vi "Dashboard Main.vi"() -> ()   [LabVIEW 2023]
uses:
  <vilib>/event_ctls.llb/eventvkey.ctl
  <vilib>/Rock Robotics/Network Tables/NT Read Numeric Array.vi
  <vilib>/Rock Robotics/Network Tables/NT Read Boolean.vi
  <vilib>/Rock Robotics/WPI/Dashboard/WPI_DashboardLogging Global.vi
panel:
  in  "Camera Settings Right":T1={"Frame Rate"=30, "Compression"=30, "Size"=1, "DB Camera Config"=FALSE} {"Frame Rate" scale=1.0..30.0; "Compression" scale=100.0..-1.0; "Size" items=["640x480", "320x240", "160x120"]}
  in  "Camera Name Right":string(combo)="No Camera Selection"
  out "Camera Perf":string
  in  "Camera Settings":T1={"Frame Rate"=30, "Compression"=30, "Size"=1, "DB Camera Config"=FALSE} {"Frame Rate" scale=1.0..30.0; "Compression" scale=100.0..-1.0; "Size" items=["640x480", "320x240", "160x120"]}
  in  "TCP":refnum<k5>
  in  "Rec Mode":enum32{"Stop", "Record", "Playback"}(radio)
  out "Robot IP":string
  out "Image Message":string="Timeout in Camera Communications"
  in  "Dashboard Tab":T2(tab)
  in  "Select Auto":string(combo)="Select Autonomous ..."
  out "NT Connection":bool
  out "MotorChart R":cluster{"Numeric":dbl, "Numeric":dbl}(graph)
  out "MotorChart L":cluster{"Numeric":dbl, "Numeric":dbl}(graph)
  out "MotorSliders R":cluster{"MotorSlide1":dbl, "MotorSlide2":dbl} {"MotorSlide2" scale=-1.0..1.0 scale format="%#_2e"; "MotorSlide1" scale=-1.0..1.0 scale format="%#_2e"}
  out "MotorSliders L":cluster{"MotorSlide1":dbl, "MotorSlide2":dbl} {"MotorSlide2" scale=-1.0..1.0 scale format="%#_2e"; "MotorSlide1" scale=-1.0..1.0 scale format="%#_2e"}
  out "Gyro":dbl(knob) scale=0.0..360.0
  out "JS1 Z":dbl(slide) scale=-1.0..1.0 scale format="%#_2e"
  out "JS1 Graph":cluster{"X":dbl, "Y":dbl}[](graph)
  out "JS1 Buttons":T3
  out "JS2 Z":dbl(slide) scale=-1.0..1.0 scale format="%#_2e"
  out "JS2 Graph":cluster{"X":dbl, "Y":dbl}[](graph)
  out "JS2 Buttons":T3
  out "Mode":T4(ring)=enum."Auto Disabled"
  out "Right Camera Perf":cluster{"Bandwidth (Mbps)":dbl, "FPS":dbl}
  out "Camera Image Right":T5(plugin-control)
  in  "DB/String 9":string
  in  "DB/String 8":string
  in  "DB/String 7":string
  in  "DB/String 6":string
  in  "DB/String 5":string
  in  "DB/String 4":string
  in  "DB/String 3":string
  in  "DB/String 2":string
  in  "DB/String 1":string
  in  "DB/String 0":string
  in  "DB/Slider 0":dbl(slide) scale=0.0..5.0
  in  "DB/Slider 1":dbl(slide) scale=0.0..5.0
  in  "DB/Slider 2":dbl(slide) scale=0.0..5.0
  in  "DB/Slider 3":dbl(slide) scale=0.0..5.0
  out "DB/LED 3":bool
  out "DB/LED 2":bool
  out "DB/LED 1":bool
  out "DB/LED 0":bool
  in  "DB/Button 3":bool
  in  "DB/Button 2":bool
  in  "DB/Button 1":bool
  in  "DB/Button 0":bool caption="New Name"
  out "Shoot Motor Out R":dbl format="%14.3f"
  out "Shoot PV RPM R":dbl format="%14.0f"
  in  "Shoot  SP RPM":dbl min=-5000.0 max=5000.0 step=200.0 format="%14.0f"
  out "Shoot Control R":T6(graph)
  out "Shoot Speed On Targ L":bool
  out "Shoot Speed On Targ R":bool
  out "Shoot PV RPM L":dbl format="%14.0f"
  out "Shoot Motor Out L":dbl format="%14.3f"
  out "Intake Motor Out":dbl format="%14.3f"
  out "Intake PV RPM":dbl format="%14.0f"
  in  "Intake  SP PCT":dbl min=-1.0 max=1.0 step=0.05 format="%14.3f"
  out "Intake Control":T7(graph)
  in  "Test Slider":dbl(slide) scale=0.0..100.0 scale format="%#_3g"
  in  "On/Off":bool caption="Solenoid"
  in  "Test Name":u16(ring) items=["Select the test to run..."]
  in  "Test Tree":string(tree)
  in  "Motor":cluster{"Value":dbl, "Enable":bool} {"Value" scale=-1.0..1.0 scale format="%#_3g"}
  out "Progress":T8 {"Test Progress" scale=0.0..100.0}
  in  "Rev/Fwd":cluster{"Forward":bool, "Reverse":bool}
  in  "Test Ring":u16(ring) items=["Monochrome", "Color"]
  in  "CheckList":i32(listbox)
  out "Tree":string(tree)
  out "Camera Image":T5(plugin-control)
  out "Background":bool
  in  "Camera Name":string(combo)="No Camera Selection"
  # "HW"
  # "HW"
  # "Joysticks"
  # "Drive Motors"
  # "Front"
  # "Right"
  # "Left"
  # "Back"
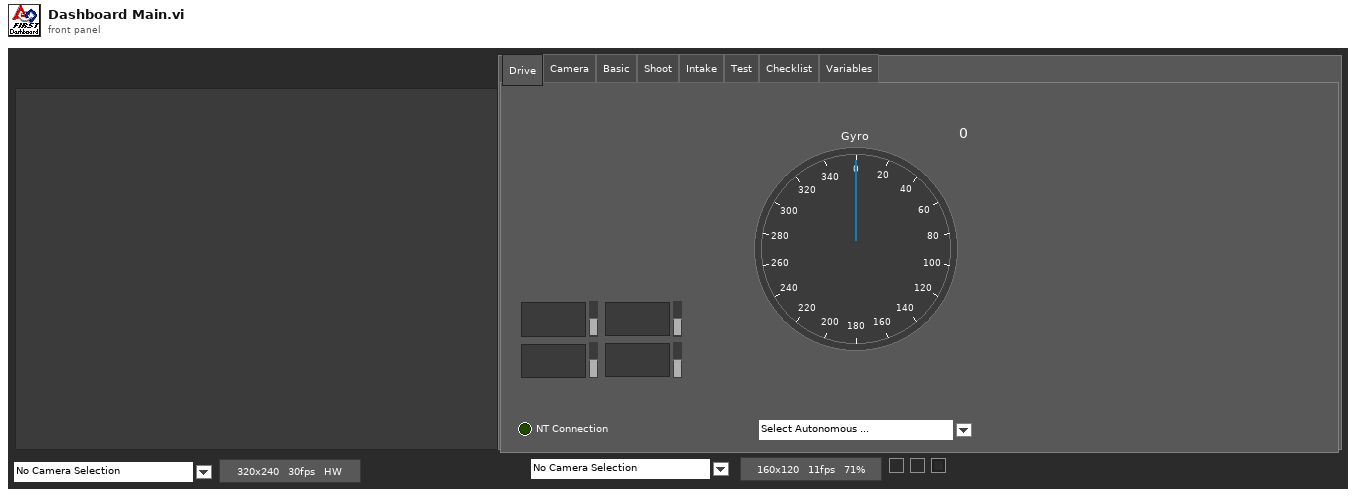
[diagram p1: front panel]
types:
  T1 = cluster{"Frame Rate":i32, "Compression":i32, "Size":u16, "DB Camera Config":bool}
  T2 = enum32{"Drive", "Camera", "Basic", "Shoot", "Intake", "Test", "Checklist", "Variables"}
  T3 = cluster{bool, bool, bool, bool, bool, bool, bool, bool, bool, bool, bool, bool}
  T4 = enum8{"Tele-Op Disabled", "Tele-Op Enabled", "Auto Disabled", "Auto Enabled", "Test Disabled", "Test Enabled", "Disconnected", "No Code", "E-Stop"}
  T5 = typedef "IMAQ Image.ctl" = refnum<image>
  T6 = cluster{"Setpoint":dbl, "FeedForward":dbl, "CO-ControlOutput":dbl, "Velocity_RPM":dbl}
  T7 = cluster{"Intake  SP PCT":dbl, "value":dbl, "value":dbl, "value":dbl}
  T8 = cluster{"Test Progress":u8, "Test Progress Text":string}
  T9 = cluster{"Save Path":path, "Interval (s)":dbl, "Keep":i32}
  T10 = enum32{"Drive", "Camera", "Basic", "Custom", "Test", "Commands", "Checklist", "Variables"}
  T11 = typedef "Image Type" = u32
  T12 = cluster{"Error Strings":string, "Disable Counts":cluster{u16, u16}, "Rail Faults":cluster{u16, u16, u16}, "Robot IP":string, "DB Mode":u8, "Event Info":cluster{"Name":string, "Type":u8, "Number":u16, "Replay":u8}}
  T13 = cluster{"Storage":cluster{"Disk Free":u64, "RAM Block":u32, "RAM free":u32}, "CPU Utilization":cluster{"CPU % ISR":sgl, "CPU % Time Crit":sgl, "CPU % Timed Str":sgl, "CPU % High":sgl, "CPU % Above":sgl, "CPU % Normal":sgl, "CPU % Low":sgl}, "CAN":cluster{"% Bus Utilization":sgl, "Bus Off Cnt":u32, "TX_FIFO Full Cnt":u32, "Receive Error Cnt":u8, "Transmit Error Cnt":u8}, "HID":cluster{"HID Outputs":u32, "Rumble Low":u16, "Rumble High":u16}[]}
  T14 = cluster{"Status bits":cluster{"Test Mode":bool, "Autonomous":bool, "Enabled":bool, "Code Start":bool, "Brownout":bool, "Reserved 2":bool, "Reserved 3":bool, "E-Stop":bool}, "Code Trace":cluster{"Disabled":bool, "TeleOp":bool, "Auto":bool, "Test":bool}, "Controller Type":enum16{"unknown", "cRIO", "roboRio"}, "Code?":enum16{"unknown", "noCode", "code"}, "Battery V":dbl}
  T15 = cluster{"Control Bits":cluster{"TestMode":bool, "Autonomous":bool, "Enabled":bool, "FMS Present":bool, bool, bool, bool, "E-Stop":bool}, "Team Station ":u8, "Countdown":sgl, "Joystick Values":cluster{"Axes":dbl[], "Buttons":bool[], "POVs":i16[]}[]}
  T16 = cluster{"Axes":dbl[], "Buttons":bool[], "POVs":i16[]}[]
  T17 = cluster{"Axes":dbl[], "Buttons":bool[], "POVs":i16[]}
  T18 = cluster{"Buttons[0]":bool, "Buttons[1]":bool, "Buttons[2]":bool, "Buttons[3]":bool, "Buttons[4]":bool, "Buttons[5]":bool, "Buttons[6]":bool, "Buttons[7]":bool, "Buttons[8]":bool, "Buttons[9]":bool, "Buttons[10]":bool, "Buttons[11]":bool}
  T19 = cluster{"Intake  SP PCT":dbl, dbl, "value":dbl, "value":dbl}
  T20 = cluster{"Shoot  SP RPM":dbl, "value":dbl, "value":dbl, "value":dbl}
  T21 = cluster{"Camera Image":refnum<vi>, "Dashboard Tab":refnum<vi>, "Background":refnum<vi>, "Rec Mode":refnum<vi>, "Test Slider":refnum<vi>, "On/Off ":refnum<vi>, "Test Ring":refnum<vi>, "Rev/Fwd":refnum<vi>, "Test Name":refnum<vi>, "Motor":refnum<vi>, "Progress":refnum<vi>, "CheckList":refnum<vi>, "Tree":refnum<vi>, "Test Tree":refnum<vi>, "Camera Settings":refnum<vi>, "Camera Name":refnum<vi>, "Camera Perf":refnum<vi>, "Camera Settings Right":refnum<vi>, "Camera Name Right":refnum<vi>, "Camera Image Right":refnum<vi>}
  T22 = cluster{"Global Rectangle":i32[], "Contours":cluster{"Contour Type":u32, "ROI Type":u32, "Points":i32[]}[]}
  T23 = cluster{"Camera Name":string, string, "Saved DB Images Info":cluster{"Save Path":path, "Interval (s)":dbl, "Keep":i32}}
  T24 = cluster{"Camera Name Right":string, string, "Saved DB Images Info":cluster{"Save Path":path, "Interval (s)":dbl, "Keep":i32}}
  T25 = cluster{"Operation":enum16{"Update", "Clear"}, "Color Box":u32}[]
  T26 = typedef "eventvkey.ctl" = enum16{"ASCII", "Enter", "Return", "Shift", "Ctrl", "Alt", "Cmd", "Opt", "Caps", "NumLock", "Clear", "Break", "Up", "Down", "Left", "Right", "Insert", "Delete", "Home", "End", "PageUp", "PageDown", "Escape", "Help", "Pause", "ScrollLock", "F1", "F2", "F3", "F4", "F5", "F6", "F7", "F8", "F9", "F10", "F11", "F12", "F13", "F14", "F15", "F16", "F17", "F18", "F19", "F20", "F21", "F22", "F23", "F24", "Play", "VolumeUp", "VolumeDown", "Mute", "Two Byte Char"}
  T27 = cluster{"Image Size":bool, "Image Type":bool, "Pixel Value":bool, "ROI Information":bool, "Zoom Factor":bool}
  T28 = cluster{"Operation":enum16{"Update", "Clear"}, "Color Box":u32}
  T29 = cluster{"Shift":bool, "Ctrl":bool, "Alt":bool, "Cmd":bool, "Opt":bool}
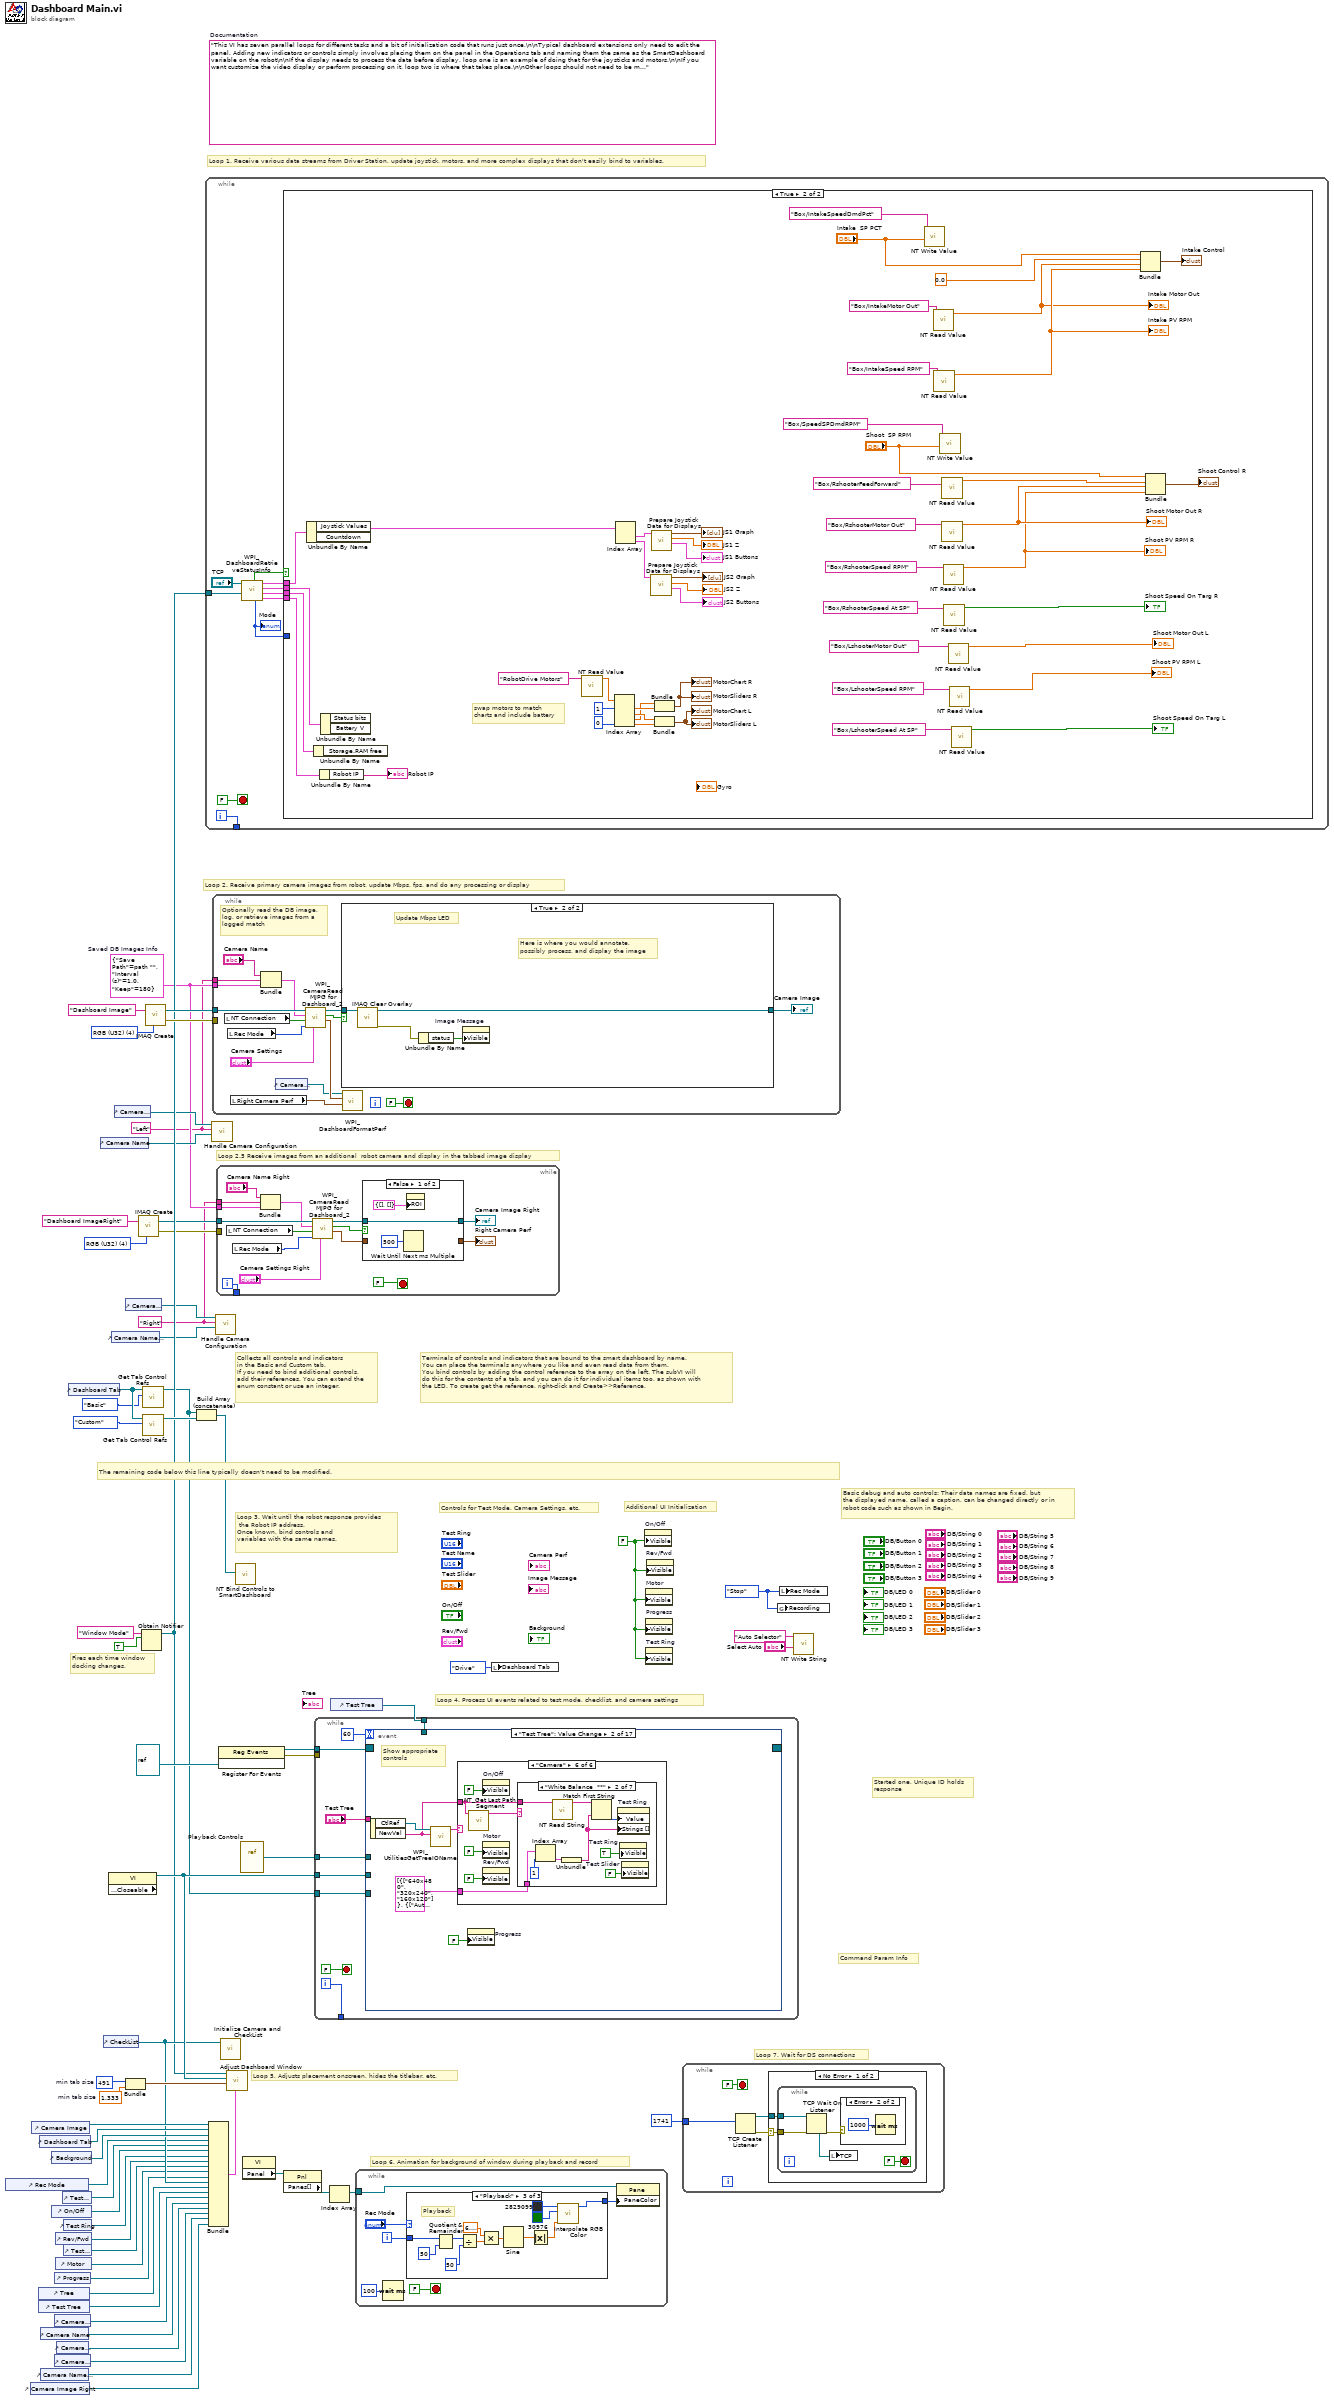
[diagram p0: block diagram]
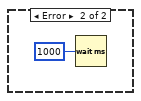
[diagram p4: hidden frame]
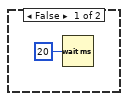
[diagram p5: hidden frame]
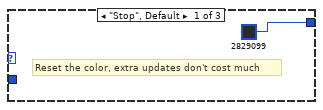
[diagram p6: hidden frame]
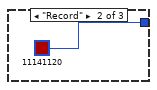
[diagram p7: hidden frame]
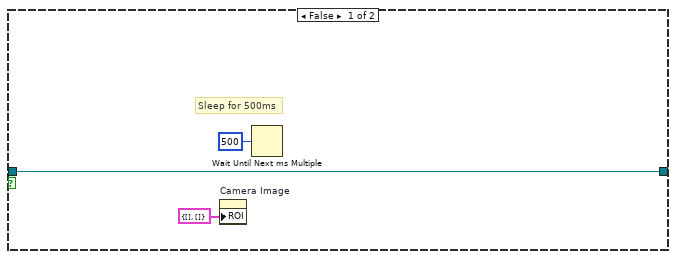
[diagram p8: hidden frame]
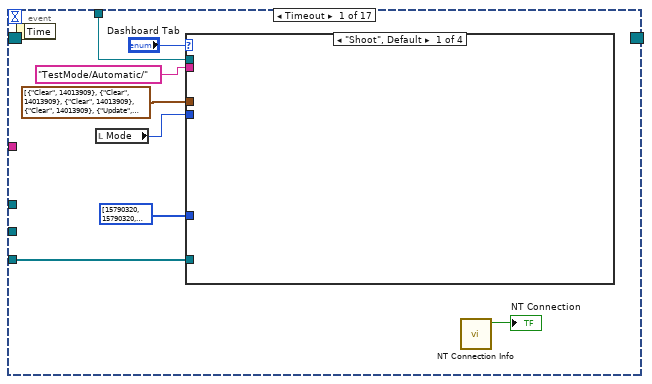
[diagram p9: hidden frame]
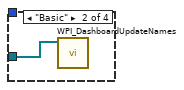
[diagram p10: hidden frame]
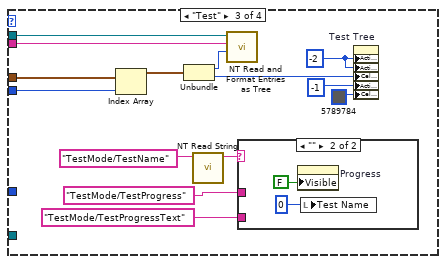
[diagram p11: hidden frame]
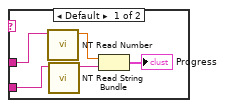
[diagram p12: hidden frame]
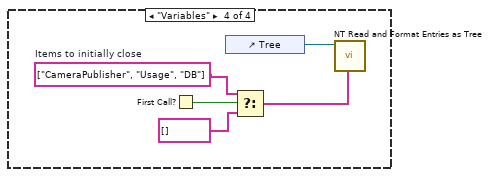
[diagram p13: hidden frame]
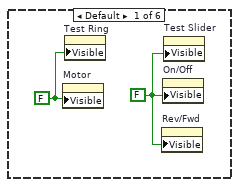
[diagram p14: hidden frame]
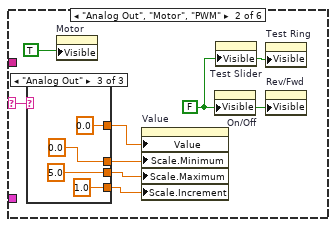
[diagram p15: hidden frame]
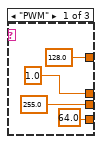
[diagram p16: hidden frame]
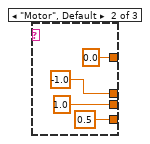
[diagram p17: hidden frame]
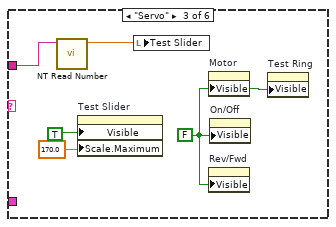
[diagram p18: hidden frame]
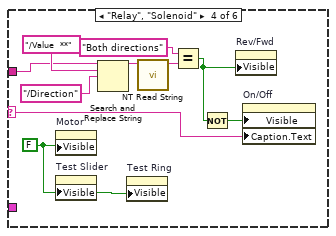
[diagram p19: hidden frame]
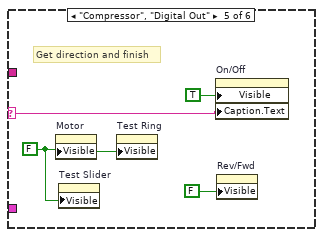
[diagram p20: hidden frame]
diagram:
  w4 = T9 {"Save Path"=path "", "Interval (s)"=1.0, "Keep"=180}  # Saved DB Images Info
  w3 = "Right"
  w2 = "Left"
  w14 = T11 4 items=["Grayscale (U8)", "Grayscale (I16)", "Grayscale (SGL)", "Complex (CSG)", "RGB (U32)", "HSL (U32)", "RGB (U64)"] ("Image Type")
  w42 = 491  # min tab size
  w41 = 1.333  # min tab size
  w49 = enum32{"Stop", "Record", "Playback"}."Stop" ("Rec Mode")
  w26 = FALSE ("Visible")
  (unwired) "This VI has seven parallel loops for different tasks and a bit of initialization code that runs just once.\n\nTypical dashboard extensions only need to edit the panel. Adding new indicators or controls simply involves placing them on the panel in the Operations tab and naming them the same as the SmartDashboard variable on the robot\n\nIf the display needs to process the data before display, loop one is an example of doing that for the joysticks and motors.\n\nIf you want customize the video display or perform processing on it, loop two is where that takes place.\n\nOther loops should not need to be modified. They are pretty standard, and document the task they perform."  # Documentation
  w63 = T11 4 items=["Grayscale (U8)", "Grayscale (I16)", "Grayscale (SGL)", "Complex (CSG)", "RGB (U32)", "HSL (U32)", "RGB (U64)"] ("Image Type")
  # "Loop 2.5 Receive images from an additional  robot camera and display in the tabbed image display"
  # "Command Param Info"
  # "Started one, Unique ID holds\nresponse"
  # "Loop 7. Wait for DS connections"
  # "Basic debug and auto controls: Their data names are fixed, but\nthe displayed name, called a caption, can be changed directly or in\nrobot code such as shown in Begin."
  # "Controls for Test Mode, Camera Settings, etc."
  # "Additional UI Initialization"
  # "Loop 6. Animation for background of window during playback and record"
  # "Fires each time window\ndocking changes."
  # "Collects all controls and indicators\nin the Basic and Custom tab.\nIf you need to bind additional controls,\nadd their references. You can extend the\nenum constant or use an integer."
  # "The remaining code below this line typically doesn't need to be modified."
  # "Loop 4. Process UI events related to test mode, checklist, and camera settings"
  # "Terminals of controls and indicators that are bound to the smart dashboard by name.\nYou can place the terminals anywhere you like and even read data from them.\nYou bind controls by adding the control reference to the array on the left. The subVI will\ndo this for the contents of a tab, and you can do it for individual items too, as shown with\nthe LED. To create get the reference, right-click and Create>>Reference."
  # "Loop 3. Wait until the robot response provides\n the Robot IP address.\nOnce known, bind controls and\nvariables with the same names."
  # "Loop 5. Adjusts placement onscreen, hides the titlebar, etc."
  # "Loop 1. Receive various data streams from Driver Station, update joystick, motors, and more complex displays that don't easily bind to variables."
  # "Loop 2. Receive primary camera images from robot, update Mbps, fps, and do any processing or display"
  n1 = control-ref of="Rec Mode"() -> (w32:refnum<vi>)
  n2 = control-ref of="Camera Image Right"() -> (w7:refnum<vi>)
  n3 = control-ref of="Camera Image"() -> (w44:refnum<vi>)
  n4 = control-ref of="Tree"() -> (w36:refnum<vi>)
  n5 = control-ref of="Test Tree"() -> (w35:refnum<vi>)
  n6 = control-ref of="Dashboard Tab"() -> (w43:refnum<vi>)
  n7 = control-ref of="Camera Name"() -> (w20:refnum<vi>)
  n8 = control-ref of="Camera Name Right"() -> (w8:refnum<vi>)
  n9 = control-ref of="Background"() -> (w39:refnum<vi>)
  n10 = control-ref of="On/Off"() -> (w30:refnum<vi>)
  n11 = control-ref of="Progress"() -> (w27:refnum<vi>)
  n12 = control-ref of="Camera Settings"() -> (w21:refnum<vi>)
  n13 = control-ref of="Camera Settings Right"() -> (w9:refnum<vi>)
  n14 = control-ref of="Rev/Fwd"() -> (w28:refnum<vi>)
  n15 = control-ref of="Motor"() -> (w33:refnum<vi>)
  n16 = control-ref of="Camera Perf"() -> (w19:refnum<vi>)
  n17 = control-ref of="Test Slider"() -> (w31:refnum<vi>)
  n18 = control-ref of="Test Ring"() -> (w29:refnum<vi>)
  n19 = control-ref of="Test Name"() -> (w34:refnum<vi>)
  n20 = control-ref of="Dashboard Tab"() -> (w47:refnum<vi>)
  n21 = control-ref of="Camera Name"() -> (w22:refnum<vi>)
  n22 = control-ref of="CheckList"() -> (w37:refnum<vi>)
  n23 = property class="VI" props=["Front Panel.Closeable"]() -> (reference out=w48:refnum<vi>)  [unwired: 2 in, 2 out]
  n24 = control-ref of="Camera Name Right"() -> (w10:refnum<vi>)
  n25 = control-ref of="Camera Settings"() -> (w23:refnum<vi>)
  n26 = control-ref of="Camera Settings Right"() -> (w11:refnum<vi>)
  n27 = Bundle("min tab size"=w42, "min tab size"=w41) -> (w40:cluster{"min tab size":i32, "min tab size":dbl})  [unwired: 1 in]
  n28 = call "IMAQ Create"("Image Name"="Dashboard ImageRight", "Image Type"=w14) -> ("New Image"=w13:T5, "error out"=w12:errorcluster)  [unwired: 2 in, 1 out]
  n29 = Obtain Notifier(name (unnamed)="Window Mode", notification data type=TRUE) -> (notifier out=w25:refnum<notifier>)  [unwired: 2 in, 2 out]
  n30 = call <vilib>:"Get Tab Control Refs.vi"("Page Index"=T10."Basic" ("Dashboard Tab"), "TabControl in"=w47) -> ("ControlsOnPage"=w18:refnum<vi>[])  [unwired: 9 in]
  n31 = call <vilib>:"Get Tab Control Refs.vi"("Page Index"=T10."Custom" ("Dashboard Tab"), "TabControl in"=w47) -> ("ControlsOnPage"=w46:refnum<vi>[])  [unwired: 9 in]
  n32 = call "IMAQ Create"("Image Name"="Dashboard Image", "Image Type"=w63) -> ("New Image"=w61:T5, "error out"=w60:errorcluster)  [unwired: 2 in, 1 out]
  n33 = Build Array (concatenate)(w18, w46) -> (w45:refnum<vi>[])
  n34 = while {
    tunnel: [w72] -> _
    tunnel: w25 -> [w64]
    i -> [w72]
    stop <- FALSE stop-if-true
    n35 = call <vilib>:"WPI_DashboardRetrieveStatusInfo.vi"("Window Mode Notifier"=w64, "TCP Cnx"="TCP") -> ("Power and Errors"=w67:T12, "Robot Metrics"=w70:T13, "Status Info"=w71:T14, "Control Info"=w68:T15, "Robot Mode"=w66:T4, "Process?"=w69:bool)  [unwired: 4 in]
    "Mode" <- w66
    n36 = case shown="True" w69 {
      tunnel: w71 -> [_ w123]
      tunnel: w70 -> [_ w122]
      tunnel: w68 -> [_ w121]
      tunnel: w67 -> [_ w120]
      tunnel: w66 -> [_ _]
      frame False {
        n37 = Wait (ms)(milliseconds to wait=u32 20) -> ()  [unwired: 1 out]
      }
      frame True {
        # "swap motors to match\ncharts and include battery"
        n38 = Unbundle By Name(w121) -> ("Joystick Values"=w111:T16)  [unwired: 1 out]
        n39 = Unbundle By Name(w122) -> ()  [unwired: 1 out]
        n40 = Unbundle By Name(w120) -> ("Robot IP"=→"Robot IP":string)
        n41 = Unbundle By Name(w123) -> ()  [unwired: 2 out]
        n42 = call-poly <vilib>:"NT Read Value.vi"("name"="RobotDrive Motors" ("Name")) -> ("value"=w101:dbl[])  [unwired: 8 in, 2 out]
        n43 = Index Array(array=w101, index #1=1, index #4=0) -> (element #1=w115:dbl, element #2=w116:dbl, element #3=w114:dbl, element #4=w119:dbl)  [unwired: 2 in]
        n44 = Index Array(array=w111) -> (element #1=w110:T17, element #2=w106:T17)  [unwired: 2 in]
        n45 = call "Prepare Joystick Data for Displays.vi"("Joystick Values"=w106) -> ("Buttons"=→"JS2 Buttons":T18, "Z Axis"=→"JS2 Z":dbl, "Cartesian Data"=→"JS2 Graph":cluster{"X axis":dbl, "X axis":dbl}[])  [unwired: 8 in]
        n46 = call "Prepare Joystick Data for Displays.vi"("Joystick Values"=w110) -> ("Buttons"=→"JS1 Buttons":T18, "Z Axis"=→"JS1 Z":dbl, "Cartesian Data"=→"JS1 Graph":cluster{"X axis":dbl, "X axis":dbl}[])  [unwired: 8 in]
        n47 = Bundle("Numeric"=w114, "Numeric"=w115) -> (→"MotorChart R" →"MotorSliders R":cluster{"Numeric":dbl, "Numeric":dbl})  [unwired: 1 in]
        n48 = Bundle("Numeric"=w116, "Numeric"=w119) -> (→"MotorChart L" →"MotorSliders L":cluster{"Numeric":dbl, "Numeric":dbl})  [unwired: 1 in]
        n49 = call-poly <vilib>:"NT Write Value.vi"("value"="Intake  SP PCT", "name"="Box/IntakeSpeedDmdPct") -> ()  [unwired: 9 in, 1 out]
        n50 = call-poly <vilib>:"NT Read Value.vi"("name"="Box/IntakeMotor Out") -> ("value"=w75:dbl)  [unwired: 8 in, 2 out]
        "Intake Motor Out" <- w75
        n51 = call-poly <vilib>:"NT Read Value.vi"("name"="Box/IntakeSpeed RPM") -> ("value"=w97:dbl)  [unwired: 8 in, 2 out]
        "Intake PV RPM" <- w97
        n52 = call-poly <vilib>:"NT Write Value.vi"("value"="Shoot  SP RPM", "name"="Box/SpeedSPDmdRPM") -> ()  [unwired: 9 in, 1 out]
        n53 = call-poly <vilib>:"NT Read Value.vi"("name"="Box/RshooterFeedForward") -> ("value"=w95:dbl)  [unwired: 8 in, 2 out]
        n54 = call-poly <vilib>:"NT Read Value.vi"("name"="Box/RshooterMotor Out") -> ("value"=w94:dbl)  [unwired: 8 in, 2 out]
        "Shoot Motor Out R" <- w94
        n55 = call-poly <vilib>:"NT Read Value.vi"("name"="Box/RshooterSpeed RPM") -> ("value"=w93:dbl)  [unwired: 8 in, 2 out]
        "Shoot PV RPM R" <- w93
        n56 = call-poly <vilib>:"NT Read Value.vi"("name"="Box/RshooterSpeed At SP") -> ("value"=→"Shoot Speed On Targ R":bool)  [unwired: 8 in, 2 out]
        n57 = call-poly <vilib>:"NT Read Value.vi"("name"="Box/LshooterMotor Out") -> ("value"=→"Shoot Motor Out L":dbl)  [unwired: 8 in, 2 out]
        n58 = call-poly <vilib>:"NT Read Value.vi"("name"="Box/LshooterSpeed RPM") -> ("value"=→"Shoot PV RPM L":dbl)  [unwired: 8 in, 2 out]
        n59 = call-poly <vilib>:"NT Read Value.vi"("name"="Box/LshooterSpeed At SP") -> ("value"=→"Shoot Speed On Targ L":bool)  [unwired: 8 in, 2 out]
        n60 = Bundle("Intake  SP PCT"="Intake  SP PCT", 0.0, "value"=w75, "value"=w97) -> (→"Intake Control":T19)  [unwired: 1 in]
        n61 = Bundle("Shoot  SP RPM"="Shoot  SP RPM", "value"=w95, "value"=w94, "value"=w93) -> (→"Shoot Control R":T20)  [unwired: 1 in]
      }
    }
  }
  n62 = Bundle("Camera Image"=w44, "Dashboard Tab"=w43, "Background"=w39, "Rec Mode"=w32, "Test Slider"=w31, "On/Off"=w30, "Test Ring"=w29, "Rev/Fwd"=w28, "Test Name"=w34, "Motor"=w33, "Progress"=w27, "CheckList"=w37, "Tree"=w36, "Test Tree"=w35, "Camera Settings"=w21, "Camera Name"=w20, "Camera Perf"=w19, "Camera Settings Right"=w9, "Camera Name Right"=w8, "Camera Image Right"=w7) -> (w38:T21)  [unwired: 1 in]
  n63 = call "Handle Camera Configuration.vi"("CameraNameRef"=w22, "Display Name"=w2, "ClusterRef"=w23) -> ()  [unwired: 9 in]
  n64 = while {
    tunnel: w61 -> [w137]
    tunnel: w60 -> [_]
    tunnel: w4 -> [w130]
    tunnel: w2 -> [w127]
    stop <- FALSE stop-if-true
    # "Optionally read the DB image,\nlog, or retrieve images from a\nlogged match"
    n65 = local read "NT Connection"() -> (w131:bool)
    n66 = local read "Rec Mode"() -> (w134:enum32{"Stop", "Record", "Playback"})
    n67 = local read "Right Camera Perf"() -> (w125:cluster{"Bandwidth (Mbps)":dbl, "FPS":dbl})
    n68 = Bundle("Camera Name"="Camera Name", w127, "Saved DB Images Info"=w130) -> (w129:T23)  [unwired: 1 in]
    n69 = control-ref of="Camera Perf"() -> (w124:refnum<vi>)
    n70 = call <vilib>:"WPI_CameraRead MJPG for Dashboard_2.vi"("Camera Settings"="Camera Settings", "Rec Mode"=w134, "NT Connection"=w131, "Capture Info"=w129, "Image in"=w137) -> ("perf info"=w126:cluster{"Bandwidth (Mbps)":dbl, "fps":dbl}, "Active"=w135:bool, "Image\\ out"=w136:T5)  [unwired: 4 in]
    n71 = case shown="True" w135 {
      tunnel: w136 -> [w140 w143]
      tunnel: [w140 w142] -> w132
      frame False {
        # "Sleep for 500ms"
        n72 = property on="Camera Image" class="ImageControl"("ROI"=T22 {"Global Rectangle"=[], "Contours"=[]}) -> ()  [unwired: 2 in, 2 out]
        n73 = Wait Until Next ms Multiple(millisecond multiple=u32 500) -> ()  [unwired: 1 out]
      }
      frame True {
        # "Here is where you would annotate,\npossibly process, and display the image"
        # "Update Mbps LED"
        n74 = call "IMAQ Clear Overlay"("Image"=w143) -> ("error out"=w144:errorcluster, "Image Out"=w142:T5)  [unwired: 2 in, 7 out]
        n75 = Unbundle By Name(w144) -> ("status"=w145:bool)
        n76 = property on="Image Message" class="Str"("Visible"=w145) -> ()  [unwired: 2 in, 2 out]
      }
    }
    "Camera Image" <- w132
    n77 = call <vilib>:"WPI_DashboardFormatPerf.vi"("Right Camera Perf"=w125, "Performance"=w126, "String in"=w124) -> ()  [unwired: 9 in]
  }
  n78 = call "Handle Camera Configuration.vi"("CameraNameRef"=w10, "Display Name"=w3, "ClusterRef"=w11) -> ()  [unwired: 9 in]
  n79 = while {
    tunnel: w13 -> [w160]
    tunnel: w12 -> [_]
    tunnel: [w155] -> _
    tunnel: w4 -> [w151]
    tunnel: w3 -> [w148]
    i -> [w155]
    stop <- FALSE stop-if-true
    n80 = local read "NT Connection"() -> (w152:bool)
    n81 = local read "Rec Mode"() -> (w159:enum32{"Stop", "Record", "Playback"})
    n82 = Bundle("Camera Name Right"="Camera Name Right", w148, "Saved DB Images Info"=w151) -> (w150:T24)  [unwired: 1 in]
    n83 = call <vilib>:"WPI_CameraRead MJPG for Dashboard_2.vi"("Camera Settings"="Camera Settings Right", "Rec Mode"=w159, "NT Connection"=w152, "Capture Info"=w150, "Image in"=w160) -> ("perf info"=w146:cluster{"Bandwidth (Mbps)":dbl, "fps":dbl}, "Active"=w154:bool, "Image\\ out"=w157:T5)  [unwired: 4 in]
    n84 = case shown="False" w154 {
      tunnel: w157 -> [w162 w165]
      tunnel: [w162 w165] -> w153
      tunnel: [_ w164] -> w147
      tunnel: w146 -> [_ w164]
      frame False {
        n85 = Wait Until Next ms Multiple(millisecond multiple=u32 500) -> ()  [unwired: 1 out]
        n86 = property on="Camera Image Right" class="ImageControl"("ROI"=T22 {"Global Rectangle"=[], "Contours"=[]}) -> ()  [unwired: 2 in, 2 out]
      }
      frame True {
      }
    }
    "Camera Image Right" <- w153
    "Right Camera Perf" <- w147
  }
  n87 = register-events(refnum<vi> refnum) -> (reference out=w52:refnum<event-registration>, error out=w51:errorcluster)  [unwired: 2 in]
  n88 = call "Initialize Camera and CheckList.vi"("ListBox in"=w37) -> ()  [unwired: 11 in]
  n89 = call "Adjust Dashboard Window.vi"("Sizing Refnums"=w38, "Size Constraints"=w40, "VI"=w48, "WIn Mode"=w25) -> ()  [unwired: 8 in]
  n90 = call <vilib>:"NT Bind Controls to SmartDashboard.vi"("Bound Control Refs"=w45) -> ()  [unwired: 11 in]
  n91 = vi-ref "Playback Controls.vi"() -> (w53:refnum<vi>)
  n92 = property class="VI"() -> ("Panel"=w55:refnum<vi>)  [unwired: 2 in, 2 out]
  n93 = property class="Pnl"(reference=w55) -> ("Panes[]"=w56:refnum<vi>[])  [unwired: 1 in, 2 out]
  n94 = Index Array(array=w56) -> (element=w54:refnum<vi>)  [unwired: 1 in]
  n95 = control-ref of="Test Tree"() -> (w57:refnum<vi>)
  n96 = while {
    tunnel: [w171] -> _
    tunnel: w57 -> [w170]
    tunnel: w53 -> [w169]
    tunnel: w52 -> [w168]
    tunnel: w51 -> [_]
    tunnel: w48 -> [w167]
    tunnel: w18 -> [w166]
    i -> [w171]
    stop <- FALSE stop-if-true
    n97 = event shown="[1] \"Test Tree\": Value Change" {
      selector: w168 -> [_ _ _ _ _ _ _ _ _ _ _ _ _ _ _ _ _]
      dyn-events: [_ _ _ _ _ _ _ _ _ _ _ _ _ w376 _ _ _] -> _
      timeout: u32 60 ("milliseconds to wait") -> [_ _ _ _ _ _ _ _ _ _ _ _ _ _ _ _ _]
      tunnel: w170 -> [w181 _ _ _ _ _ _ _ _ _ _ _ _ _ _ _ _]
      tunnel: "Test Tree" -> [_ _ _ _ _ _ _ _ w349 w356 w357 w360 w367 _ _ _ _]
      tunnel: w169 -> [_ _ _ _ _ _ _ _ _ _ _ _ _ w378 _ w393 _]
      tunnel: w167 -> [_ _ _ _ _ _ _ _ _ _ _ _ _ w374 _ _ _]
      tunnel: w166 -> [w176 _ _ _ _ _ _ _ _ _ _ _ _ _ _ _ _]
      event Timeout {
        n98 = event-data() -> ()  [unwired: 1 in, 1 out]
        n99 = local read "Mode"() -> (w179:T4)
        n100 = case shown="\"Shoot\", Default" "Dashboard Tab" {
          tunnel: w181 -> [_ _ w197 _]
          tunnel: "TestMode/Automatic/" ("Name Pattern") -> [_ _ w196 _]
          tunnel: T25 [{"Operation"=enum."Clear", "Color Box"=14013909}, {"Operation"=enum."Clear", "Color Box"=14013909}, {"Operation"=enum."Clear", "Color Box"=14013909}, {"Operation"=enum."Clear", "Color Box"=14013909}, {"Operation"=enum."Update", "Color Box"=14013909}, {"Operation"=enum."Update", "Color Box"=16777215}, {"Operation"=enum."Clear", "Color Box"=14013909}, {"Operation"=enum."Clear", "Color Box"=14013909}, {"Operation"=enum."Clear", "Color Box"=14013909}] -> [_ _ w189 _]
          tunnel: w179 -> [_ _ w188 _]
          tunnel: u32[] [15790320, 15790320, 15790320, 15790320, 16777215, 16777215, 15790320, 15790320, 15790320] -> [_ _ _ _]
          tunnel: w176 -> [_ w183 _ _]
          frame "Shoot", Default {
          }
          frame "Basic" {
            n101 = call <vilib>:"WPI_DashboardUpdateNames.vi"("Controls on Tab"=w183) -> ()  [unwired: 11 in]
          }
          frame "Test" {
            w195 = -2 ("Active Item:Row Number")
            n102 = Index Array(array=w189, index=w188) -> (element=w190:T28)
            n103 = Unbundle(w190) -> ("Operation"=w191:enum16{"Update", "Clear"}, "Color Box"=w192:u32)
            n104 = call <vilib>:"NT Read String.vi"("name"="TestMode/TestName" ("Name")) -> ("value"=w186:string)  [unwired: 8 in, 2 out]
            n105 = call <vilib>:"NT Read and Format Entries as Tree.vi"("Operation"=w191, "Name Pattern"=w196, "Tree Refnum"=w197) -> ()  [unwired: 7 in, 2 out]
            n106 = case shown="\"\"" w186 {
              tunnel: "TestMode/TestProgress" ("Name") -> [w199 _]
              tunnel: "TestMode/TestProgressText" ("Name") -> [w198 _]
              frame Default {
                n107 = call <vilib>:"NT Read Number.vi"("name"=w199) -> ("value"=w200:dbl)  [unwired: 8 in, 2 out]
                n108 = call <vilib>:"NT Read String.vi"("name"=w198) -> ("value"=w201:string)  [unwired: 8 in, 2 out]
                n109 = Bundle("value"=w200, "value"=w201) -> (→"Progress":cluster{"value":dbl, "value":string})  [unwired: 1 in]
              }
              frame "" {
                n110 = property on="Progress" class="Clust (strict)"("Visible"=FALSE) -> ()  [unwired: 2 in, 2 out]
                n111 = local write "Test Name"(u16 0) -> ()
              }
            }
            n112 = property on="Test Tree" class="Tree (strict)"("Active Item Row Number"=w195, "ActiveColNum"=w195, "CellBG"=w192, "Active Item Row Number"=-1 ("Active Item:Row Number"), "CellBG"=u32 5789784 ("Color Box")) -> ()  [unwired: 2 in, 2 out]
          }
          frame "Variables" {
            w207 = string[] ["CameraPublisher", "Usage", "DB"]  # Items to initially close
            n113 = First Call?() -> (First Call?: T/F=w208:bool)
            n114 = control-ref of="Tree"() -> (w209:refnum<vi>)
            n115 = Select(t=w207, s=w208, f=string[] []) -> (s? t:f=w205:string[])
            n116 = call <vilib>:"NT Read and Format Entries as Tree.vi"("Tags to  Close"=w205, "Tree Refnum"=w209) -> ()  [unwired: 8 in, 2 out]
          }
        }
        n117 = call <vilib>:"NT Connection Info.vi"() -> ("Connected"=→"NT Connection":bool)  [unwired: 11 in]
      }
      event "Test Tree": Value Change {
        # "Show appropriate\ncontrols"
        n118 = event-data() -> ("CtlRef"=w213:refnum<vi>, "NewVal"=w211:string)  [unwired: 1 in]
        n119 = call <vilib>:"WPI_UtilitiesGetTreeIOName.vi"("NewVal"=w211, "TreeControl in"=w213) -> ("I/O Name"=w214:string)  [unwired: 9 in]
        n120 = case shown="\"Camera\"" w214 {
          selector: w214 -> [_ w221 _ w243 w252 _]
          tunnel: w211 -> [_ _ w240 w242 _ w259]
          tunnel: cluster{string[]}[] [{["640x480", "320x240", "160x120"]}, {["Auto", "Fixed indoor", "Fixed outdoor 1", "Fixed outdoor 2", "Fixed fluorescent 1", "Fixed fluorescent 2", "Hold current"]}, {["Auto", "Flicker-free 50 Hz", "Flicker-free 60 Hz", "Hold current"]}, {["None", "Prioritize frame rate", "Prioritize image quality"]}, {["Monochrome", "Color"]}] -> [_ _ _ _ _ w258]
          frame Default {
            w216 = FALSE ("Visible")
            w215 = FALSE ("Visible")
            n121 = property on="Motor" class="Clust (strict)"("Visible"=w215) -> ()  [unwired: 2 in, 2 out]
            n122 = property on="Test Ring" class="Ring (strict)"("Visible"=w215) -> ()  [unwired: 2 in, 2 out]
            n123 = property on="Rev/Fwd" class="Clust (strict)"("Visible"=w216) -> ()  [unwired: 2 in, 2 out]
            n124 = property on="On/Off" class="Bool (strict)"("Visible"=w216) -> ()  [unwired: 2 in, 2 out]
            n125 = property on="Test Slider" class="Slide (strict)"("Visible"=w216) -> ()  [unwired: 2 in, 2 out]
          }
          frame "Analog Out", "Motor", "PWM" {
            w222 = FALSE ("Visible")
            n126 = case shown="\"Analog Out\"" w221 {
              tunnel: [1.0 ("Value") -1.0 ("Value") 0.0 ("Value")] -> w220
              tunnel: [255.0 ("Value") 1.0 ("Value") 5.0 ("Value")] -> w219
              tunnel: [128.0 ("Value") 0.0 ("Value") 0.0 ("Value")] -> w218
              tunnel: [64.0 ("Value") 0.5 ("Value") 1.0 ("Value")] -> w217
              frame "PWM" {
              }
              frame "Motor", Default {
              }
              frame "Analog Out" {
              }
            }
            n127 = property on="Motor" class="Clust (strict)"("Visible"=TRUE) -> ()  [unwired: 2 in, 2 out]
            n128 = property on="Value" class="Slide (strict)"("Value"=w218, "Scale.Minimum"=w220, "Scale.Maximum"=w219, "Scale.Increment"=w217) -> ()  [unwired: 2 in, 2 out]
            n129 = property on="On/Off" class="Bool (strict)"("Visible"=w222) -> ()  [unwired: 2 in, 2 out]
            n130 = property on="Test Slider" class="Slide (strict)"("Visible"=w222) -> ()  [unwired: 2 in, 2 out]
            n131 = property on="Test Ring" class="Ring (strict)"("Visible"=w222) -> ()  [unwired: 2 in, 2 out]
            n132 = property on="Rev/Fwd" class="Clust (strict)"("Visible"=w222) -> ()  [unwired: 2 in, 2 out]
          }
          frame "Servo" {
            w238 = FALSE ("Visible")
            n133 = call <vilib>:"NT Read Number.vi"("name"=w240) -> ("value"=w239:dbl)  [unwired: 8 in, 2 out]
            n134 = property on="Test Slider" class="Slide (strict)"("Visible"=TRUE, "Scale.Maximum"=170.0 ("Scale.Range:Maximum")) -> ()  [unwired: 2 in, 2 out]
            n135 = local write "Test Slider"(w239) -> ()
            n136 = property on="Motor" class="Clust (strict)"("Visible"=w238) -> ()  [unwired: 2 in, 2 out]
            n137 = property on="Rev/Fwd" class="Clust (strict)"("Visible"=w238) -> ()  [unwired: 2 in, 2 out]
            n138 = property on="On/Off" class="Bool (strict)"("Visible"=w238) -> ()  [unwired: 2 in, 2 out]
            n139 = property on="Test Ring" class="Ring (strict)"("Visible"=w238) -> ()  [unwired: 2 in, 2 out]
          }
          frame "Relay", "Solenoid" {
            w241 = FALSE ("Visible")
            n140 = property on="Motor" class="Clust (strict)"("Visible"=w241) -> ()  [unwired: 2 in, 2 out]
            n141 = property on="Test Slider" class="Slide (strict)"("Visible"=w241) -> ()  [unwired: 2 in, 2 out]
            n142 = Search and Replace String(input string=w242, search string="/Value  **", replace string="/Direction") -> (result string=w248:string)  [unwired: 5 in, 3 out]
            n143 = property on="Test Ring" class="Ring (strict)"("Visible"=w241) -> ()  [unwired: 2 in, 2 out]
            n144 = call <vilib>:"NT Read String.vi"("name"=w248) -> ("value"=w246:string)  [unwired: 8 in, 2 out]
            n145 = Equal?(x="Both directions", y=w246) -> (x = y?=w244:bool)
            n146 = Not(x=w244) -> (.not. x?=w245:bool)
            n147 = property on="Rev/Fwd" class="Clust (strict)"("Visible"=w244) -> ()  [unwired: 2 in, 2 out]
            n148 = property on="On/Off" class="Bool (strict)"("Visible"=w245, "Caption.Text"=w243) -> ()  [unwired: 2 in, 2 out]
          }
          frame "Compressor", "Digital Out" {
            w251 = FALSE ("Visible")
            # "Get direction and finish"
            n149 = property on="Motor" class="Clust (strict)"("Visible"=w251) -> ()  [unwired: 2 in, 2 out]
            n150 = property on="Test Slider" class="Slide (strict)"("Visible"=w251) -> ()  [unwired: 2 in, 2 out]
            n151 = property on="Test Ring" class="Ring (strict)"("Visible"=w251) -> ()  [unwired: 2 in, 2 out]
            n152 = property on="On/Off" class="Bool (strict)"("Visible"=TRUE, "Caption.Text"=w252) -> ()  [unwired: 2 in, 2 out]
            n153 = property on="Rev/Fwd" class="Clust (strict)"("Visible"=FALSE) -> ()  [unwired: 2 in, 2 out]
          }
          frame "Camera" {
            n154 = call <vilib>:"NT_Get Last Path Segment.vi"("String in"=w259) -> ("String out"=w260:string)  [unwired: 10 in]
            n155 = property on="On/Off" class="Bool (strict)"("Visible"=FALSE) -> ()  [unwired: 2 in, 2 out]
            n156 = property on="Motor" class="Clust (strict)"("Visible"=FALSE) -> ()  [unwired: 2 in, 2 out]
            n157 = property on="Rev/Fwd" class="Clust (strict)"("Visible"=FALSE) -> ()  [unwired: 2 in, 2 out]
            n158 = case shown="\"White Balance  **\"" w260 {
              tunnel: w259 -> [w266 w275 w284 w293 w302 _ w308]
              tunnel: w258 -> [w264 w272 w281 w290 w299 _ _]
              frame "Size  **" {
                n159 = Index Array(array=w264) -> (element=w263:cluster{string[]})  [unwired: 1 in]
                n160 = call <vilib>:"NT Read String.vi"("name"=w266) -> ("value"=w265:string)  [unwired: 8 in, 2 out]
                n161 = Unbundle(w263) -> (w261:string[])
                n162 = Match First String(2:w261, 3:w265) -> (0:w262:i32)  [unwired: 1 out]
                n163 = property on="Test Ring" class="Ring (strict)"("Value"=w262, "Strings []"=w261) -> ()  [unwired: 2 in, 2 out]
                n164 = property on="Test Ring" class="Ring (strict)"("Visible"=TRUE) -> ()  [unwired: 2 in, 2 out]
                n165 = property on="Test Slider" class="Slide (strict)"("Visible"=FALSE) -> ()  [unwired: 2 in, 2 out]
              }
              frame "White Balance  **" {
                n166 = Index Array(array=w272, index=1) -> (element=w273:cluster{string[]})
                n167 = call <vilib>:"NT Read String.vi"("name"=w275) -> ("value"=w274:string)  [unwired: 8 in, 2 out]
                n168 = Unbundle(w273) -> (w270:string[])
                n169 = Match First String(2:w270, 3:w274) -> (0:w269:i32)  [unwired: 1 out]
                n170 = property on="Test Ring" class="Ring (strict)"("Value"=w269, "Strings []"=w270) -> ()  [unwired: 2 in, 2 out]
                n171 = property on="Test Ring" class="Ring (strict)"("Visible"=TRUE) -> ()  [unwired: 2 in, 2 out]
                n172 = property on="Test Slider" class="Slide (strict)"("Visible"=FALSE) -> ()  [unwired: 2 in, 2 out]
              }
              frame "Exposure  **" {
                n173 = Index Array(array=w281, index=2) -> (element=w282:cluster{string[]})
                n174 = call <vilib>:"NT Read String.vi"("name"=w284) -> ("value"=w283:string)  [unwired: 8 in, 2 out]
                n175 = Unbundle(w282) -> (w278:string[])
                n176 = Match First String(2:w278, 3:w283) -> (0:w279:i32)  [unwired: 1 out]
                n177 = property on="Test Ring" class="Ring (strict)"("Value"=w279, "Strings []"=w278) -> ()  [unwired: 2 in, 2 out]
                n178 = property on="Test Ring" class="Ring (strict)"("Visible"=TRUE) -> ()  [unwired: 2 in, 2 out]
                n179 = property on="Test Slider" class="Slide (strict)"("Visible"=FALSE) -> ()  [unwired: 2 in, 2 out]
              }
              frame "Exposure Priority  **" {
                n180 = Index Array(array=w290, index=3) -> (element=w291:cluster{string[]})
                n181 = call <vilib>:"NT Read String.vi"("name"=w293) -> ("value"=w292:string)  [unwired: 8 in, 2 out]
                n182 = Unbundle(w291) -> (w287:string[])
                n183 = Match First String(2:w287, 3:w292) -> (0:w288:i32)  [unwired: 1 out]
                n184 = property on="Test Ring" class="Ring (strict)"("Value"=w288, "Strings []"=w287) -> ()  [unwired: 2 in, 2 out]
                n185 = property on="Test Ring" class="Ring (strict)"("Visible"=TRUE) -> ()  [unwired: 2 in, 2 out]
                n186 = property on="Test Slider" class="Slide (strict)"("Visible"=FALSE) -> ()  [unwired: 2 in, 2 out]
              }
              frame "Color Enable  **" {
                n187 = Index Array(array=w299, index=4) -> (element=w300:cluster{string[]})
                n188 = call <vilib>:"NT Read String.vi"("name"=w302) -> ("value"=w301:string)  [unwired: 8 in, 2 out]
                n189 = Unbundle(w300) -> (w296:string[])
                n190 = Match First String(2:w296, 3:w301) -> (0:w297:i32)  [unwired: 1 out]
                n191 = property on="Test Ring" class="Ring (strict)"("Value"=w297, "Strings []"=w296) -> ()  [unwired: 2 in, 2 out]
                n192 = property on="Test Ring" class="Ring (strict)"("Visible"=TRUE) -> ()  [unwired: 2 in, 2 out]
                n193 = property on="Test Slider" class="Slide (strict)"("Visible"=FALSE) -> ()  [unwired: 2 in, 2 out]
              }
              frame Default {
                n194 = property on="Test Ring" class="Ring (strict)"("Visible"=FALSE) -> ()  [unwired: 2 in, 2 out]
                n195 = property on="Test Slider" class="Slide (strict)"("Visible"=FALSE) -> ()  [unwired: 2 in, 2 out]
              }
              frame "Brightness  **", "Color Level  **", "Compression  **", "FPS  **", "Sharpness  **" {
                n196 = call <vilib>:"NT Read Number.vi"("name"=w308) -> ("value"=w307:dbl)  [unwired: 8 in, 2 out]
                n197 = local write "Test Slider"(w307) -> ()
                n198 = property on="Test Ring" class="Ring (strict)"("Visible"=FALSE) -> ()  [unwired: 2 in, 2 out]
                n199 = property on="Test Slider" class="Slide (strict)"("Visible"=TRUE, "Scale.Maximum"=100.0 ("Scale.Range:Maximum")) -> ()  [unwired: 2 in, 2 out]
              }
            }
          }
        }
        n200 = property on="Progress" class="Clust (strict)"("Visible"=FALSE) -> ()  [unwired: 2 in, 2 out]
      }
      event "Test Name": Mouse Enter {
        # "Populate the ring with the list of tests"
        n201 = event-data() -> ()  [unwired: 1 in, 1 out]
        n202 = call <vilib>:"NT Read String Array.vi"("name"="TestMode/TestList" ("Name")) -> ("value"=w315:string[])  [unwired: 8 in, 2 out]
        n203 = Build Array (concatenate)("Select the test to run...", w315) -> (w314:string[])
        n204 = property on="Test Name" class="Ring (strict)"("Strings []"=w314) -> ()  [unwired: 2 in, 2 out]
      }
      event "Test Name": Value Change {
        w316 = FALSE ("Visible")
        # "Tell the robot the test name to run"
        n205 = event-data() -> ("NewVal"=w320:u16)  [unwired: 1 in]
        n206 = property on="Test Name" class="Ring (strict)"() -> ("Strings []"=w321:string[])  [unwired: 2 in, 2 out]
        n207 = local write "Progress"(T8 {"Test Progress"=0, "Test Progress Text"=""} ("Progress")) -> ()
        n208 = Index Array(array=w321, index=w320) -> (element=w319:string)
        n209 = call <vilib>:"NT Write String.vi"("value"=w319, "name"="TestMode/TestName" ("Name")) -> ()  [unwired: 9 in, 1 out]
        n210 = property on="Progress" class="Clust (strict)"("Visible"=TRUE) -> ()  [unwired: 2 in, 2 out]
        n211 = property on="Motor" class="Clust (strict)"("Visible"=w316) -> ()  [unwired: 2 in, 2 out]
        n212 = property on="Test Slider" class="Slide (strict)"("Visible"=w316) -> ()  [unwired: 2 in, 2 out]
        n213 = property on="On/Off" class="Bool (strict)"("Visible"=w316) -> ()  [unwired: 2 in, 2 out]
        n214 = property on="Rev/Fwd" class="Clust (strict)"("Visible"=w316) -> ()  [unwired: 2 in, 2 out]
        n215 = property on="Test Ring" class="Ring (strict)"("Visible"=w316) -> ()  [unwired: 2 in, 2 out]
      }
      event "Select Auto": Mouse Enter {
        # "Populate the combo box with the list of autonomous options"
        n216 = event-data() -> ()  [unwired: 1 in, 1 out]
        n217 = call <vilib>:"NT Read String Array.vi"("name"="Auto List" ("Name")) -> ("value"=w323:string[])  [unwired: 8 in, 2 out]
        n218 = property on="Select Auto" class="CmbBox"("Strings[]"=w323) -> ()  [unwired: 2 in, 2 out]
      }
      event "Select Auto": Value Change {
        # "User modified the Auto Selection. Write to NT variable so robot knows."
        n219 = event-data() -> ("NewVal"=w325:string)  [unwired: 1 in]
        n220 = call <vilib>:"NT Write String.vi"("value"=w325, "name"="Auto Selector" ("Name")) -> ()  [unwired: 9 in, 1 out]
      }
      event "CheckList": Double Click {
        # "Shift clears all"
        # "Update symbols on the listbox"
        n221 = event-data() -> ("PlatMods.Shift"=w327:bool, "Row"=w329:i32)  [unwired: 1 in]
        n222 = case shown="True" w327 {
          tunnel: w329 -> [w333 _]
          tunnel: 1 -> [w332 _]
          frame False {
            n223 = property on="CheckList" class="LstBox (strict)"() -> ("Item Symbols"=w331:i32[])  [unwired: 2 in, 2 out]
            n224 = Replace Array Subset(array=w331, new element=w332, index=w333) -> (w330:i32[])
            n225 = property on="CheckList" class="LstBox (strict)"("Item Symbols"=w330) -> ()  [unwired: 2 in, 2 out]
          }
          frame True {
            w334 = 0 ("Top Row")
            n226 = property on="CheckList" class="LstBox (strict)"() -> ("Number of Rows"=w336:u32)  [unwired: 2 in, 2 out]
            n227 = Initialize Array(0, w336) -> (w335:i32[])
            n228 = property on="CheckList" class="LstBox (strict)"("Top Row"=w334, "Value"=w334, "Item Symbols"=w335) -> ()  [unwired: 2 in, 2 out]
          }
        }
      }
      event "CheckList": Key Down {
        # "Update symbols on the listbox\nLeft and right keys check and uncheck"
        n229 = event-data() -> ("VKey"=w339:T26)  [unwired: 1 in]
        n230 = case shown="\"Left\", \"Right\"" w339 {
          selector: w339 -> [w344 _]
          tunnel: eventvkey."Left" ("VKey") -> [w342 _]
          frame "Left", "Right" {
            n231 = Equal?(x=w342, y=w344) -> (x = y?=w343:bool)
            n232 = Select(t=0, s=w343, f=1) -> (s? t:f=w345:i32)
            n233 = property on="CheckList" class="LstBox (strict)"() -> ("Item Symbols"=w348:i32[])  [unwired: 2 in, 2 out]
            n234 = Replace Array Subset(array=w348, new element=w345, index="CheckList") -> (w347:i32[])
            n235 = property on="CheckList" class="LstBox (strict)"("Item Symbols"=w347) -> ()  [unwired: 2 in, 2 out]
          }
          frame Default {
          }
        }
      }
      event "Motor.Enable": Value Change {
        # "When the test mode otor enable helper is set, update that\ntree row item's value"
        n236 = event-data() -> ("NewVal"=w353:bool)  [unwired: 1 in]
        n237 = Unbundle("Motor") -> ("Value"=w352:dbl)  [unwired: 1 out]
        n238 = Select(t=w352, s=w353, f=0.0) -> (s? t:f=w350:dbl)
        n239 = call <vilib>:"NT Write Number.vi"("value"=w350, "name"=w349) -> ()  [unwired: 9 in, 1 out]
      }
      event "Test Slider": Value Change {
        # "When the test mode slider helper is set, update that\ntree row item's value"
        n240 = event-data() -> ("NewVal"=w355:dbl)  [unwired: 1 in]
        n241 = call <vilib>:"NT Write Number.vi"("value"=w355, "name"=w356) -> ()  [unwired: 9 in, 1 out]
      }
      event "On/Off": Value Change {
        # "When the test mode on/off helper value is set, update that\ntree row item's value"
        n242 = event-data() -> ("NewVal"=w359:bool)  [unwired: 1 in]
        n243 = Boolean To (0,1)(Boolean=w359) -> (0, 1=w358:i16)
        n244 = call <vilib>:"NT Write Number.vi"("value"=w358, "name"=w357) -> ()  [unwired: 9 in, 1 out]
      }
      event "Rev/Fwd": Value Change {
        # "When the test mode helper value for relays is set, update that\ntree row item's value"
        n245 = event-data() -> ("NewVal.Forward"=w366:bool, "NewVal.Reverse"=w365:bool)  [unwired: 1 in]
        n246 = Boolean To (0,1)(Boolean=w366) -> (0, 1=w362:i16)
        n247 = Boolean To (0,1)(Boolean=w365) -> (0, 1=w364:i16)
        n248 = Negate(x=w364) -> (-x=w363:i16)
        n249 = Add(x=w362, y=w363) -> (x+y=w361:i16)
        n250 = call <vilib>:"NT Write Number.vi"("value"=w361, "name"=w360) -> ()  [unwired: 9 in, 1 out]
      }
      event "Test Ring": Value Change {
        # "When a test mode helper value is selected from the ring,\nset the tree item's variable to the string value"
        n251 = event-data() -> ("NewVal"=w369:u16)  [unwired: 1 in]
        n252 = property on="Test Ring" class="Ring (strict)"() -> ("Strings []"=w370:string[])  [unwired: 2 in, 2 out]
        n253 = Index Array(array=w370, index=w369) -> (element=w368:string)
        n254 = call <vilib>:"NT Write String.vi"("value"=w368, "name"=w367) -> ()  [unwired: 9 in, 1 out]
      }
      event "Rec Mode": Value Change {
        # "Update globals for recording mode and path to read log from.\nClear when logging and let NetworkTables set path for vision to\nuse."
        n255 = event-data() -> ("NewVal"=w379:enum32{"Stop", "Record", "Playback"})  [unwired: 1 in]
        n256 = global write "WPI_DashboardLogging Global.vi" "Logging Filename"(path "") -> ()
        n257 = global write "WPI_DashboardLogging Global.vi" "Recording"(w379) -> ()
        n258 = case shown="\"Playback\"" w379 {
          tunnel: w378 -> [_ w381 w389]
          tunnel: [_ _ w388] -> w376
          tunnel: [_ _ w387] -> _
          tunnel: w374 -> [_ _ w385]
          tunnel: cluster{i32, i32} {-250, 170} -> [_ _ w384]
          tunnel: [_ _ T27 {"Image Size"=TRUE, "Image Type"=TRUE, "Pixel Value"=TRUE, "ROI Information"=TRUE, "Zoom Factor"=FALSE} ("Image Information Shown:All Elements")] -> w371
          tunnel: [_ _ TRUE ("Zoom Factor")] -> w372
          frame Default {
          }
          frame "Stop", "Record" {
            # "Place Window too"
            n259 = invoke class="VI" method="FP.Close"(reference=w381) -> (reference out=w380:refnum<vi>)  [unwired: 2 in, 2 out]
            n260 = invoke class="VI" method="Abort VI"(reference=w380) -> ()  [unwired: 2 in, 3 out]
          }
          frame "Playback" {
            n261 = call "Open Playback Panel.vi"("Offset"=w384, "DB VI Ref"=w385, "Playback in"=w389) -> ("Playback out"=w386:refnum<vi>)  [unwired: 8 in]
            n262 = register-events(w386) -> (reference out=w388:refnum<event-registration>, error out=w387:errorcluster)  [unwired: 2 in]
          }
        }
        n263 = property on="Camera Image Right" class="ImageControl"("Image Information Shown"=w371, "Image Information Visible"=w372) -> ()  [unwired: 2 in, 2 out]
        n264 = property on="Camera Image" class="ImageControl"("Image Information Shown"=w371, "Image Information Visible"=w372) -> ()  [unwired: 2 in, 2 out]
        n265 = call <vilib>:"WPI_DashboardNT Log FieldName Cache.vi"("Operation"=enum16{"Lookup/Add", "Index", "Clear"}."Clear") -> ()  [unwired: 8 in, 3 out]
      }
      event Panel Close {
        w390 = enum32{"Stop", "Record", "Playback"}."Stop" ("Rec Mode")
        # "Playback window has been closed, abort"
        n266 = event-data() -> ()  [unwired: 1 in, 4 out]
        n267 = local write "Rec Mode"(w390) -> ()
        n268 = global write "WPI_DashboardLogging Global.vi" "Recording"(w390) -> ()
      }
      event Panel Close {
        # "Abort playback window and ourself"
        n269 = event-data() -> ()  [unwired: 1 in, 4 out]
        n270 = invoke class="VI" method="FP.Close"(reference=w393) -> (reference out=w392:refnum<vi>)  [unwired: 2 in, 2 out]
        n271 = invoke class="VI" method="Abort VI"(reference=w392) -> (error out=w391:errorcluster)  [unwired: 2 in, 2 out]
        n272 = invoke class="VI" method="Abort VI"(error in=w391) -> ()  [unwired: 2 in, 3 out]
      }
      event "Tree": Double Click {
        n273 = event-data() -> ("PlatMods"=w399:T29, "Tag"=w396:string)  [unwired: 1 in]
        n274 = Unbundle(w399) -> ("Shift"=w398:bool)  [unwired: 4 out]
        n275 = String Subset(string=w396, length (rest)=1 ("length (rest)")) -> (substring=w395:string)  [unwired: 1 in]
        n276 = Not(x=w398) -> (.not. x?=w397:bool)
        n277 = case shown="\"/\"" w395 {
          tunnel: w396 -> [_ w401]
          tunnel: w397 -> [_ w400]
          frame Default {
          }
          frame "/" {
            n278 = call <vilib>:"NT Update Persistence.vi"("Persistence"=w400, "Name"=w401) -> ()  [unwired: 9 in, 1 out]
          }
        }
      }
    }
  }
  n279 = while {
    tunnel: w54 -> [w403]
    i -> [w406]
    stop <- FALSE stop-if-true
    n280 = Wait (ms)(milliseconds to wait=u32 100) -> ()  [unwired: 1 out]
    n281 = case shown="\"Playback\"" "Rec Mode" {
      tunnel: w406 -> [_ _ w421]
      tunnel: [u32 2829099 ("Base Color") u32 11141120 ("Target Color") w410] -> w402
      frame "Stop", Default {
        # "Reset the color, extra updates don't cost much"
      }
      frame "Record" {
      }
      frame "Playback" {
        # "Playback"
        n282 = Quotient & Remainder(x=w421, y=u32 50 ("milliseconds to wait")) -> (x-y*floor(x/y)=w417:u32)  [unwired: 1 out]
        n283 = Divide(x=w417, y=u32 50 ("milliseconds to wait")) -> (x/y=w414:dbl)
        n284 = Multiply(x=6.283185307179586, y=w414) -> (x*y=w419:dbl)
        n285 = Sine(x=w419) -> (sin(x)=w418:dbl)
        n286 = Absolute Value(x=w418) -> (abs(x)=w411:dbl)
        n287 = call "Interpolate RGB Color.vi"("Proportion"=w411, "Target Color"=u32 30976, "Base Color"=u32 2829099) -> ("Result Color"=w410:u32)  [unwired: 8 in]
      }
    }
    n288 = property class="Pane"(reference=w403, "PaneColor"=w402) -> ()  [unwired: 1 in, 2 out]
  }
  n289 = local write "Dashboard Tab"(T2."Drive" ("Dashboard Tab")) -> ()
  n290 = property on="On/Off" class="Bool (strict)"("Visible"=w26) -> ()  [unwired: 2 in, 2 out]
  n291 = property on="Motor" class="Clust (strict)"("Visible"=w26) -> ()  [unwired: 2 in, 2 out]
  n292 = property on="Progress" class="Clust (strict)"("Visible"=w26) -> ()  [unwired: 2 in, 2 out]
  n293 = property on="Test Ring" class="Ring (strict)"("Visible"=w26) -> ()  [unwired: 2 in, 2 out]
  n294 = property on="Rev/Fwd" class="Clust (strict)"("Visible"=w26) -> ()  [unwired: 2 in, 2 out]
  n295 = while {
    tunnel: u16 1741 ("timeout ms (25000)") -> [w423]
    stop <- FALSE stop-if-true
    n296 = TCP Create Listener(10:w423) -> (0:w422:errorcluster, 3:w424:refnum<k5>)  [unwired: 4 in, 1 out]
    n297 = case shown="No Error" w422 {
      selector: w422 -> [w426 _]
      tunnel: w424 -> [w427 _]
      frame No Error {
        n298 = while {
          tunnel: w427 -> [w430]
          tunnel: w426 -> [w429]
          stop <- FALSE stop-if-true
          n299 = TCP Wait On Listener(8:w429, 11:w430) -> (0:w431:errorcluster, 4:w432:refnum<k5>)  [unwired: 2 in, 3 out]
          n300 = local write "TCP"(w432) -> ()
          n301 = case shown="Error" w431 {
            frame No Error {
            }
            frame Error {
              n302 = Wait (ms)(milliseconds to wait=u32 1000) -> ()  [unwired: 1 out]
            }
          }
        }
      }
      frame Error {
        n303 = Wait (ms)(milliseconds to wait=u32 1000) -> ()  [unwired: 1 out]
      }
    }
  }
  n304 = global write "WPI_DashboardLogging Global.vi" "Recording"(w49) -> ()
  n305 = local write "Rec Mode"(w49) -> ()
  n306 = call <vilib>:"NT Write String.vi"("value"="Select Auto", "name"="Auto Selector" ("Name")) -> ()  [unwired: 9 in, 1 out]
